vi "verification_existance.vi"(1 "num_cmd":string) -> (0 "Result Set":string[][](table) caption="Afficher la commande par son Id :")   [LabVIEW 2024]
uses:
  <vilib>/drjdpowell/SQLite Library/SQL Statement/SQL Statement.lvclass/SQL Statement.ctl
  <vilib>/drjdpowell/SQLite Library/SQL Connection/Open (string).vi
  <vilib>/drjdpowell/SQLite Library/SQL Statement/Error Message.vi
  <vilib>/drjdpowell/SQLite Library/SQL Connection/Execute SQL.vi
  <vilib>/drjdpowell/SQLite Library/SQL Connection/Connection.lvclass
  <vilib>/drjdpowell/SQLite Library/SQL Statement/SQL Statement.lvclass
  <vilib>/drjdpowell/SQLite Library/SQLite.lvlib
panel:
  out "La commamnde n'existe pas":bool[](array[boolean])
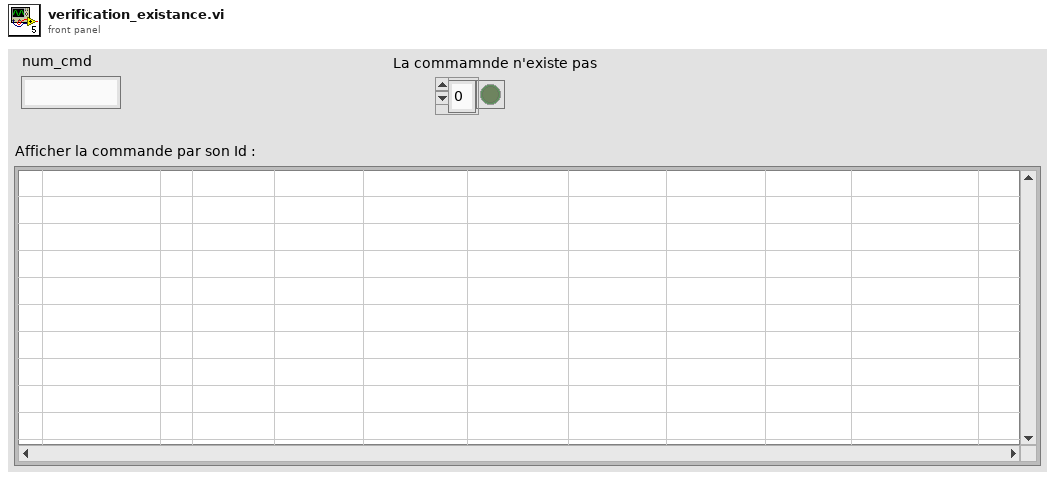
[diagram p1: front panel]
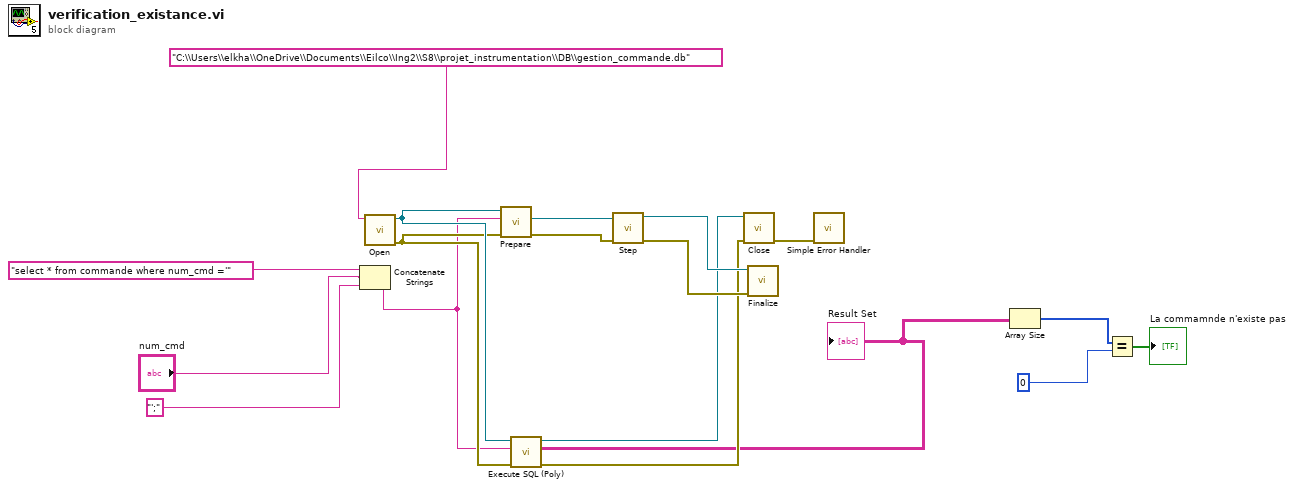
[diagram p0: block diagram]
diagram:
  n1 = Concatenate Strings("select * from commande where num_cmd ='" ("SQL"), "num_cmd", "';" ("SQL")) -> (w6:string)
  n2 = call-poly <vilib>:"Open.vi"("db file"="C:\\Users\\elkha\\OneDrive\\Documents\\Eilco\\Ing2\\S8\\projet_instrumentation\\DB\\gestion_commande.db") -> ("error out"=w10:errorcluster, "SQLite Connection"=w12:refnum<class "Connection.lvclass">)  [unwired: 9 in]
  n3 = call <vilib>:"Prepare.vi"("error in (no error)"=w10, "SQL"=w6, "SQLite Connection in"=w12) -> ("error out"=w15:errorcluster, "SQL Statement"=w16:refnum<class "SQL Statement.lvclass">)  [unwired: 4 in, 3 out]
  n4 = call-poly <vilib>:"Execute SQL (Poly).vi"("error in (no error)"=w10, "SQL"=w6, "SQLite Connection in"=w12) -> ("error out"=w9:errorcluster, "Result Set"=w4:string[][], "SQLite Connection"=w11:refnum<class "Connection.lvclass">)  [unwired: 5 in, 1 out]
  "Result Set" <- w4
  n5 = call <vilib>:"Step.vi"("error in (no error)"=w15, "SQL Statement in"=w16) -> ("error out"=w13:errorcluster, "SQL Statement"=w14:refnum<class "SQL Statement.lvclass">)  [unwired: 7 in, 1 out]
  n6 = call-dynamic "Close.vi"("error in (no error)"=w9, "SQLite Connection in"=w11) -> ("error out"=w17:errorcluster)  [unwired: 9 in]
  n7 = call <vilib>:"Finalize.vi"("error in (no error)"=w13, "SQL Statement in"=w14) -> ()  [unwired: 9 in, 1 out]
  n8 = call <vilib>:"Simple Error Handler.vi"("error in (no error)"=w17) -> ()  [unwired: 4 in, 5 out]
  n9 = Array Size(array=w4) -> (size(s)=w3:i32[])
  n10 = Equal?(x=w3, y=0) -> (x = y?=→"La commamnde n'existe pas":bool[])
